vi "Listbox Show.vi"(8 "error in (no error)":errorcluster, 11 "[V] Login in":refnum<class "[V] Login.lvclass">) -> (0 "error out":errorcluster, 3 "[V] Login out":refnum<class "[V] Login.lvclass">)   [LabVIEW 2020, in "[V] Login.lvlib" / "[V] Login.lvclass"]
uses:
  [V] Login.lvclass
  [V] Login.lvclass/[V] Login.ctl
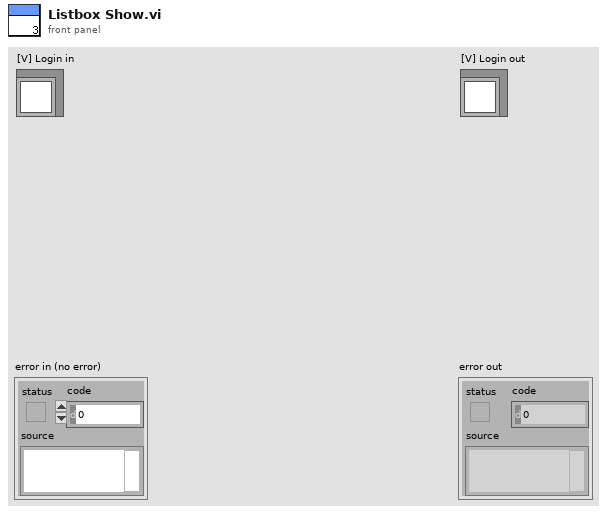
[diagram p1: front panel]
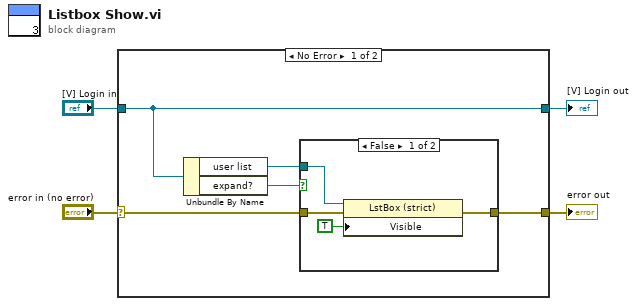
[diagram p0: block diagram]
diagram:
  n1 = case shown="No Error" "error in (no error)" {
    selector: "error in (no error)" -> [w8 w16]
    tunnel: [w6 w16] -> w3
    tunnel: [w9 w15] -> w1
    tunnel: "[V] Login in" -> [w9 w15]
    frame No Error {
      n2 = Unbundle By Name(w9) -> ("user list"=w7:refnum<vi>, "expand?"=w5:bool)
      n3 = case shown="False" w5 {
        tunnel: w8 -> [w13 w14]
        tunnel: w7 -> [w12 _]
        tunnel: [w11 w14] -> w6
        frame False {
          n4 = property class="LstBox (strict)"(reference=w12, error in=w13, "Visible"=TRUE) -> (error out=w11:errorcluster)  [unwired: 1 out]
        }
        frame True {
        }
      }
    }
    frame Error {
    }
  }
  "error out" <- w3
  "[V] Login out" <- w1
